vi "Previous_File.vi"(11 "Path in":path) -> (3 "Path out":path)   [LabVIEW 2012]
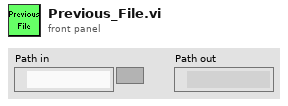
[diagram p1: front panel]
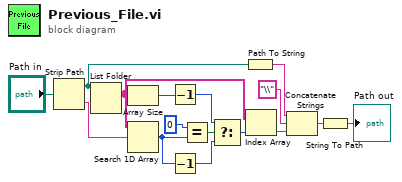
[diagram p0: block diagram]
diagram:
  n1 = Strip Path(path="Path in") -> (stripped path=w7:path, name=w3:string)
  n2 = List Folder(path=w7) -> (filenames=w10:string[])  [unwired: 3 in, 3 out]
  n3 = Array Size(array=w10) -> (size(s)=w4:i32)
  n4 = Search 1D Array(1D array=w10, element=w3) -> (index of element=w15:i32)  [unwired: 1 in]
  n5 = Decrement(x=w4) -> (x-1=w1:i32)
  n6 = Decrement(x=w15) -> (x-1=w14:i32)
  n7 = Equal?(x=0, y=w15) -> (x = y?=w13:bool)
  n8 = Select(t=w1, s=w13, f=w14) -> (s? t:f=w16:i32)
  n9 = Path To String(path=w7) -> (string=w6:string)
  n10 = Index Array(array=w10, index=w16) -> (element=w5:string)
  n11 = Concatenate Strings(w6, "\\", w5) -> (w9:string)
  n12 = String To Path(string=w9) -> (path=→"Path out":path)
